vi "UpdateDM2000English.vi"(8 "error in (no error)":errorcluster) -> (0 "error out":errorcluster, 2 "Update":bool, 3 "UpdatePath":string)   [LabVIEW 2013, in "main.lvlib"]
uses:
  main.lvlib
  <userlib>/_MGI/Error Handling/MGI Suppress Error Code/MGI Suppress Error Code (Scalar).vi
panel:
  in  "UpdateProgram":bool
  out "VersionInformationStr":string
  in  "CheckVersionsBtn":bool
  # "Update Service"
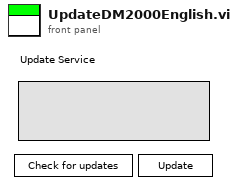
[diagram p1: front panel]
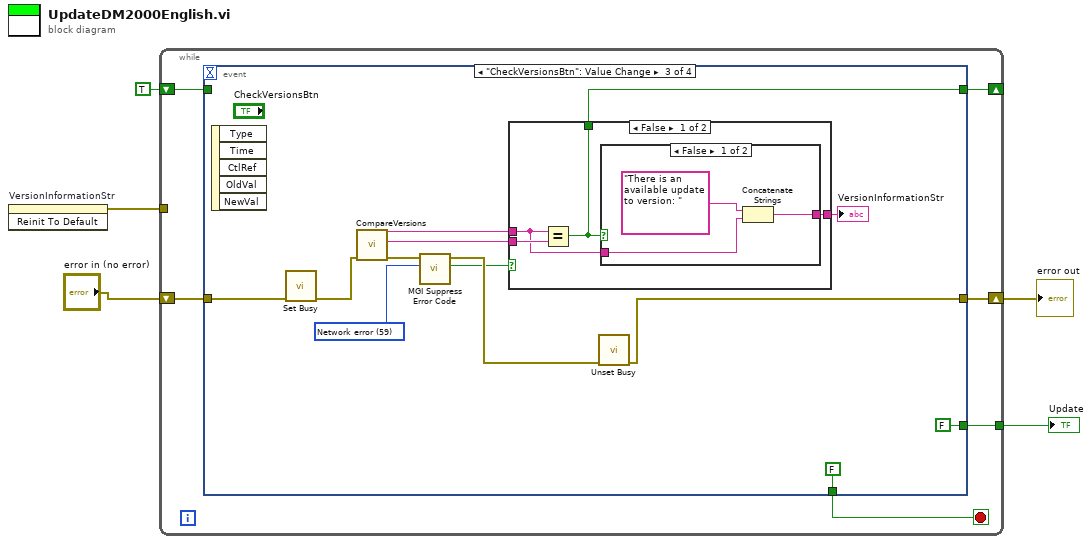
[diagram p0: block diagram]
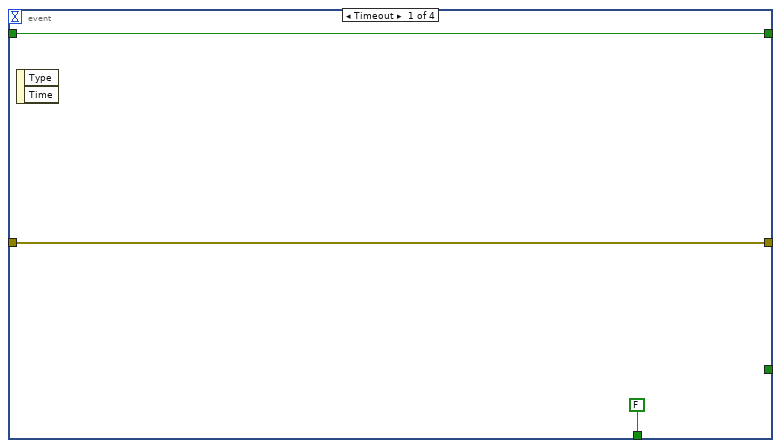
[diagram p2: hidden frame]
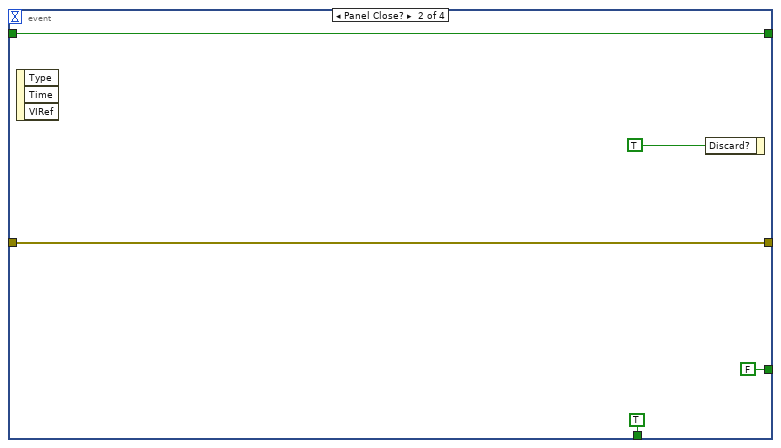
[diagram p3: hidden frame]
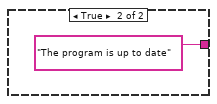
[diagram p4: hidden frame]
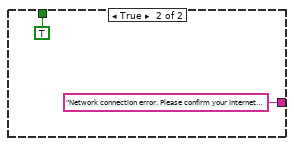
[diagram p5: hidden frame]
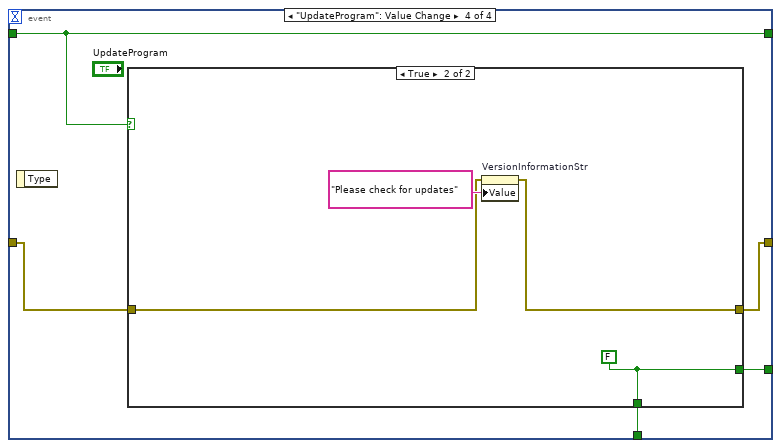
[diagram p6: hidden frame]
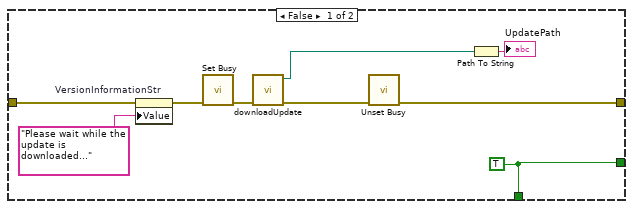
[diagram p7: hidden frame]
diagram:
  n1 = invoke on="VersionInformationStr" class="Str" method="Reinit To Default"() -> (error out=w3:errorcluster)  [unwired: 3 in, 2 out]
  n2 = while {
    shift-right: [w10] -> _
    shift-left: TRUE -> [w9]
    tunnel: [w8] -> w4
    tunnel: w3 -> [_]
    shift-right: [w6] -> w1
    shift-left: "error in (no error)" -> [w7]
    stop <- w11 stop-if-true
    n3 = event shown="[2] \"CheckVersionsBtn\": Value Change" {
      selector: _ -> [_ _ _ _]
      dyn-events: _ -> [_ _ _ _]
      timeout: _ -> [_ _ _ _]
      tunnel: [FALSE TRUE FALSE w46] -> w11
      tunnel: [w13 w17 w27 w47] -> w10
      tunnel: w9 -> [w13 w17 _ w47]
      tunnel: [_ FALSE FALSE w45] -> w8
      tunnel: w7 -> [w12 w15 w21 w44]
      tunnel: [w12 w15 w20 w43] -> w6
      event Timeout {
        n4 = event-data() -> ()  [unwired: 1 in, 2 out]
      }
      event Panel Close? {
        n5 = event-data() -> ()  [unwired: 1 in, 3 out]
        n6 = event-data("Discard?"=TRUE) -> ()  [unwired: 1 in, 1 out]
      }
      event "CheckVersionsBtn": Value Change {
        w23 = 59 items=["No error", "Argument error", "Memory is full", "Out of zone", "End of file", "File already open", "Generic file I/O error", "File not found", "File permission error", "Disk is full", "Duplicate path", "Too many files open", "System feature not enabled", "Resource file not found", "Cannot add resource", "Resource not found", "Image not found", "Image memory error", "Pen does not exist", "Config type invalid", "Config token not found", "Config parse error", "Config memory error", "Bad external code format", "Bad external code offset", "External code not present", "Null window", "Destroy window error", "Null menu", "Print aborted", "Bad print record", "Print driver error", "Windows error during printing", "Memory error during printing", "Print dialog error", "Generic print error", "Invalid device refnum", "Device not found", "Device parameter error", "Device unit error", "Cannot open device", "Device call aborted", "Generic error", "Cancelled by user", "Object ID too low", "Object ID too high", "Object not in heap", "Unknown heap", "Unknown object (invalid DefProc)", "Unknown object (DefProc not in table)", "Message out of range", "Invalid (null) method", "Unknown message", "Manager call not supported", "Bad address", "Network operation in progress", "Network operation timed out", "Connection is busy", "Network attribute not supported", "Network error", "Address in use", "System out of memory", "Connection aborted", "Connection refused", "Not connected", "Already connected", "Connection closed", "Initialization error (interapplication manager)", "Bad occurrence", "Wait on unbound occurrence handler", "Occurrence queue overflow", "Datalog type conflict", "Unused", "Unrecognized type (interapplication manager)", "Memory corrupt", "Failed to make temporary DLL", "Old CIN version", "Drag socket not found", "Failed to load drop-object", "Failed to register OLE object", "Failed to release OLE object", "Format specifier type mismatch", "Unknown format specifier", "Too few format specifiers", "Too many format specifiers", "Scan failed", "Newer CIN version", "OLE Convert", "Runtime menu error", "Password tampered", "Unknown error code"] ("Error Code")
        n7 = event-data() -> ()  [unwired: 1 in, 5 out]
        n8 = call <vilib>:"Set Busy.vi"("error in (no error)"=w21) -> ("error out"=w28:errorcluster)  [unwired: 9 in, 1 out]
        n9 = call "CompareVersions.vi"("error in (no error)"=w28) -> ("error out"=w25:errorcluster, "FileVersion"=w30:string, "Web File Version"=w29:string)  [unwired: 8 in]
        n10 = call-poly <userlib>:"MGI Suppress Error Code.vi"("Error Code"=w23, "Error In"=w25) -> ("Error Supressed?"=w22:bool, "Error Out"=w24:errorcluster)  [unwired: 4 in]
        n11 = case shown="False" w22 {
          tunnel: [w36 "Network connection error. Please confirm your internet connection"] -> w31
          tunnel: w30 -> [w35 _]
          tunnel: w29 -> [w34 _]
          tunnel: [w33 TRUE] -> w27
          frame False {
            n12 = Equal?(x=w34, y=w35) -> (x = y?=w33:bool)
            n13 = case shown="False" w33 {
              tunnel: [w39 "The program is up to date"] -> w36
              tunnel: w34 -> [w37 _]
              frame False {
                n14 = Concatenate Strings("There is an available update to version: ", w37) -> (w39:string)
              }
              frame True {
              }
            }
          }
          frame True {
          }
        }
        "VersionInformationStr" <- w31
        n15 = call <vilib>:"Unset Busy.vi"("error in (no error)"=w24) -> ("error out"=w20:errorcluster)  [unwired: 10 in]
      }
      event "UpdateProgram": Value Change {
        n16 = event-data() -> ()  [unwired: 1 in, 1 out]
        n17 = case shown="True" w47 {
          tunnel: [w53 w59] -> w46
          tunnel: [w53 w59] -> w45
          tunnel: w44 -> [w49 w58]
          tunnel: [w48 w57] -> w43
          frame False {
            w53 = TRUE
            n18 = property on="VersionInformationStr" class="Str"(error in=w49, "Value"="Please wait while the update is downloaded..." ("VersionInformationStr")) -> (error out=w55:errorcluster)  [unwired: 1 in, 1 out]
            n19 = call <vilib>:"Set Busy.vi"("error in (no error)"=w55) -> ("error out"=w52:errorcluster)  [unwired: 9 in, 1 out]
            n20 = call "downloadUpdate.vi"("error in (no error)"=w52) -> ("error out"=w50:errorcluster, "appended path"=w51:path)  [unwired: 9 in]
            n21 = call <vilib>:"Unset Busy.vi"("error in (no error)"=w50) -> ("error out"=w48:errorcluster)  [unwired: 10 in]
            n22 = Path To String(path=w51) -> (string=→"UpdatePath":string)
          }
          frame True {
            w59 = FALSE
            n23 = property on="VersionInformationStr" class="Str"(error in=w58, "Value"="Please check for updates" ("VersionInformationStr")) -> (error out=w57:errorcluster)  [unwired: 1 in, 1 out]
          }
        }
      }
    }
  }
  "Update" <- w4
  "error out" <- w1
